vi "FT10_Semi-Auto Tester.vi"(7 "Read/ Write":T9, 8 "Error In":errorcluster, 10 "Semi-Auto Cluster in":T1 {"Power Level" format="%.1f"}, 11 "Path":path=path "FT10_rev2/Semi-Auto Commands.csv") -> (0 "Error Out":errorcluster, 2 "Semi-Auto Cluster out":T1 {"Power Level" format="%.1f"}, 3 "Semi-Auto 2-D Array out":T8)   [LabVIEW 2015]
doc: "READ = read CSV at specified path and pass commands out to be executed if user chooses.\n\nWRITE = write the cluster array to the specified CSV filepath. Then pass commands out to be executed if user chooses."
uses:
  LV2024/NI Online Practice/CLD Practice/cld_success_package/Preparation_Materials/CLD 6/CLD 6 CSV file enum.ctl
  Controls/Control_Semi-Auto 2-D Array.ctl
  Controls/Control_Semi-Auto Cluster Array.ctl
  Controls/Control_Semi-Auto Cluster.ctl
  Controls/Control_Semi-Auto Unitherm Load.ctl
  Controls/Control_Semi-Auto Port.ctl
  Controls/Control_Semi-Auto Mode.ctl
  Controls/Control_Semi-Auto Power Level.ctl
  Controls/Control_Semi-Auto Activation Duration.ctl
  Controls/Control_Semi-Auto 1-D Array.ctl
  <vilib>/Utility/file.llb/Read Delimited Spreadsheet (string).vi
  <vilib>/Utility/file.llb/Write Delimited Spreadsheet (string).vi
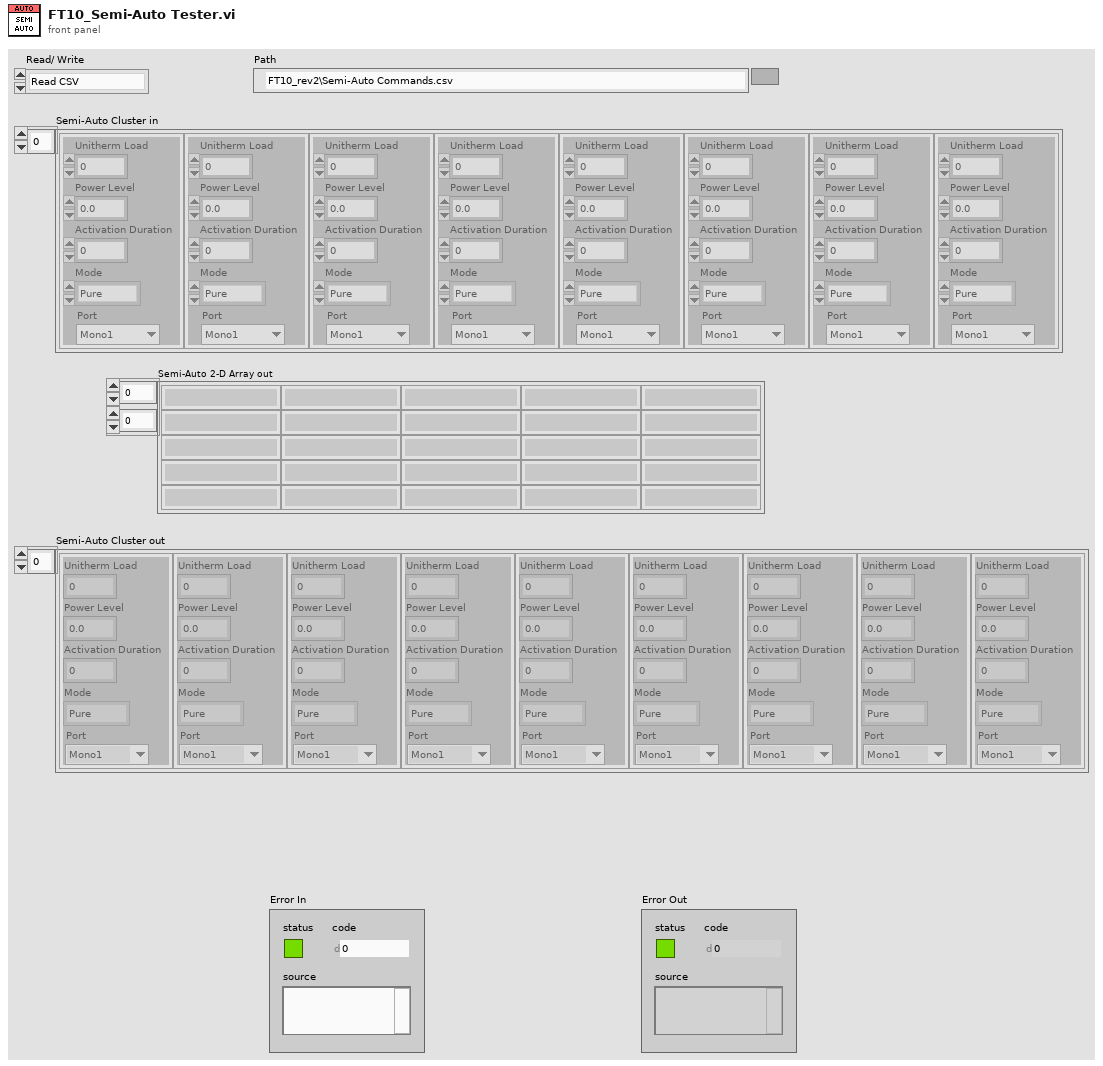
[diagram p1: front panel]
types:
  T1 = typedef "Control_Semi-Auto Cluster Array.ctl" = T2[]
  T2 = typedef "Control_Semi-Auto Cluster.ctl" = cluster{"Unitherm Load":T3, "Port":T4, "Mode":T5, "Power Level":T6, "Activation Duration":T7}
  T3 = typedef "Control_Semi-Auto Unitherm Load.ctl" = i32
  T4 = typedef "Control_Semi-Auto Port.ctl" = enum16{"Mono1", "Mono2", "Bipolar", "Ligasure", "Error"}
  T5 = typedef "Control_Semi-Auto Mode.ctl" = enum16{"Pure", "Blend", "Spray", "Fulgerate", "Standard", "Macro", "Precision", "Ligasure", "Error"}
  T6 = typedef "Control_Semi-Auto Power Level.ctl" = dbl
  T7 = typedef "Control_Semi-Auto Activation Duration.ctl" = i32
  T8 = typedef "Control_Semi-Auto 2-D Array.ctl" = string[][]
  T9 = typedef "CLD 6 CSV file enum.ctl" = enum16{"Read CSV", "Write CSV"}
  T10 = typedef "Control_Semi-Auto 1-D Array.ctl" = string[]
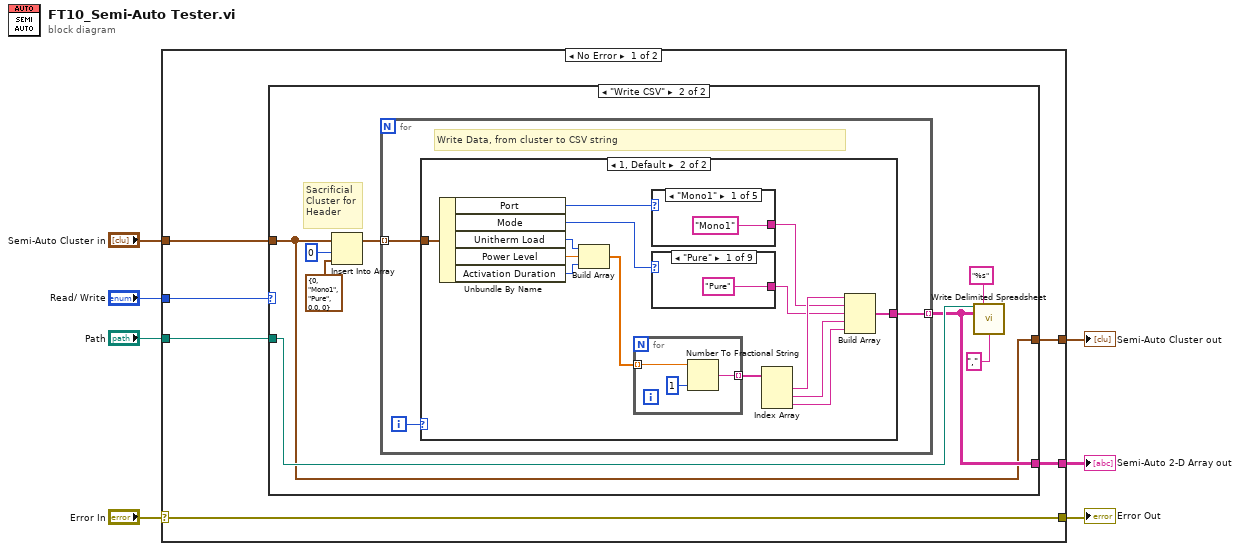
[diagram p0: block diagram]
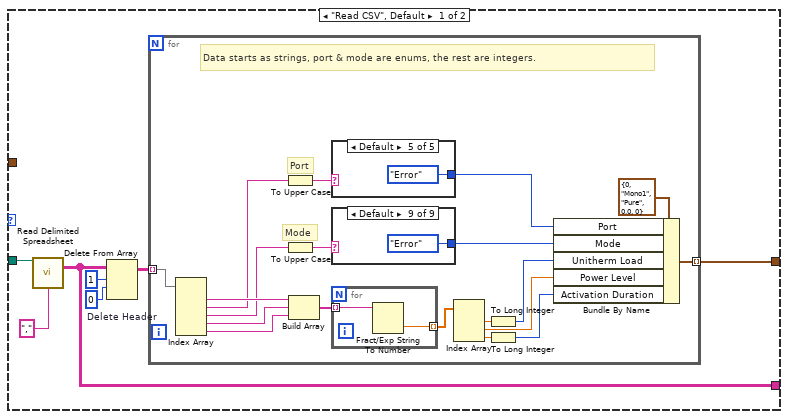
[diagram p2: hidden frame]
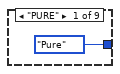
[diagram p3: hidden frame]
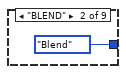
[diagram p4: hidden frame]
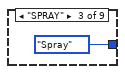
[diagram p5: hidden frame]
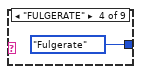
[diagram p6: hidden frame]
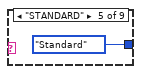
[diagram p7: hidden frame]
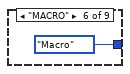
[diagram p8: hidden frame]
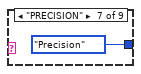
[diagram p9: hidden frame]
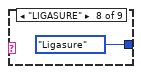
[diagram p10: hidden frame]
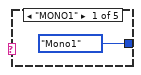
[diagram p11: hidden frame]
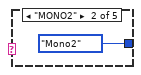
[diagram p12: hidden frame]
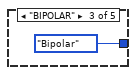
[diagram p13: hidden frame]
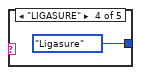
[diagram p14: hidden frame]
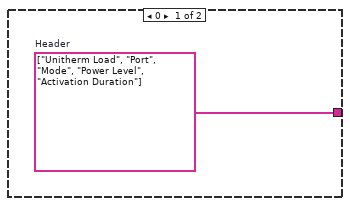
[diagram p15: hidden frame]
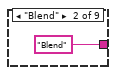
[diagram p16: hidden frame]
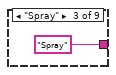
[diagram p17: hidden frame]
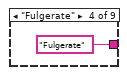
[diagram p18: hidden frame]
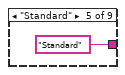
[diagram p19: hidden frame]
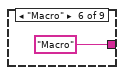
[diagram p20: hidden frame]
diagram:
  n1 = case shown="No Error" "Error In" {
    selector: "Error In" -> [w10 w101]
    tunnel: [w13 T1 []] -> w2
    tunnel: "Path" -> [w8 _]
    tunnel: "Read/ Write" -> [w12 _]
    tunnel: "Semi-Auto Cluster in" -> [w11 _]
    tunnel: [w10 w101] -> w4
    tunnel: [w9 string[][] [] ("all rows")] -> w3
    frame No Error {
      n2 = case shown="\"Write CSV\"" w12 {
        tunnel: w8 -> [w19 w62]
        tunnel: [w20 w59] -> w13
        tunnel: w11 -> [_ w59]
        tunnel: [w17 w60] -> w9
        frame "Read CSV", Default {
          n3 = call-poly <vilib>:"Read Delimited Spreadsheet.vi"("file path (dialog if empty)"=w19, "delimiter (\\t)"="," ("delimiter (\\t)")) -> ("all rows"=w17:string[][])  [unwired: 8 in, 5 out]
          n4 = Delete From Array "Delete Header"(array=w17, length=1, index (row)=0) -> (array with subset deleted=w16:string[][])  [unwired: 1 in, 1 out]
          n5 = for {
            tunnel: w16 -> [w39] mode=indexing
            tunnel: [w21] -> w20 mode=indexing
            # "Mode"
            # "Port"
            # "Data starts as strings, port & mode are enums, the rest are integers."
            n6 = Index Array "Index Array"(array=w39) -> (element #1=w38:string, element #2=w34:string, element #3=w33:string, element #4=w37:string, element #5=w36:string)  [unwired: 5 in]
            n7 = To Upper Case(1:w34) -> (0:w28:string)
            n8 = To Upper Case(1:w33) -> (0:w29:string)
            n9 = Build Array(w38, w37, w36) -> (w32:string[])
            n10 = case shown="Default" w28 {
              tunnel: [Control_Semi-Auto_Port."Mono1" ("Port") Control_Semi-Auto_Port."Mono2" ("Port") Control_Semi-Auto_Port."Bipolar" ("Port") Control_Semi-Auto_Port."Ligasure" ("Port") Control_Semi-Auto_Port."Error" ("Port")] -> w27
              frame "MONO1" {
              }
              frame "MONO2" {
              }
              frame "BIPOLAR" {
              }
              frame "LIGASURE" {
              }
              frame Default {
              }
            }
            n11 = case shown="Default" w29 {
              tunnel: [Control_Semi-Auto_Mode."Pure" ("Mode") Control_Semi-Auto_Mode."Blend" ("Mode") Control_Semi-Auto_Mode."Spray" ("Mode") Control_Semi-Auto_Mode."Fulgerate" ("Mode") Control_Semi-Auto_Mode."Standard" ("Mode") Control_Semi-Auto_Mode."Macro" ("Mode") Control_Semi-Auto_Mode."Precision" ("Mode") Control_Semi-Auto_Mode."Ligasure" ("Mode") Control_Semi-Auto_Mode."Error" ("Mode")] -> w26
              frame "PURE" {
              }
              frame "BLEND" {
              }
              frame "SPRAY" {
              }
              frame "FULGERATE" {
              }
              frame "STANDARD" {
              }
              frame "MACRO" {
              }
              frame "PRECISION" {
              }
              frame "LIGASURE" {
              }
              frame Default {
              }
            }
            n12 = for {
              tunnel: w32 -> [w55] mode=indexing
              tunnel: [w54] -> w31 mode=indexing
              n13 = Fract/Exp String To Number(string=w55) -> (number=w54:dbl)  [unwired: 3 in, 1 out]
            }
            n14 = Index Array "Index Array"(array=w31) -> (element #1=w24:dbl, element #2=w25:dbl, element #3=w30:dbl)  [unwired: 3 in]
            n15 = To Long Integer(number=w24) -> (32bit integer=w23:i32)
            n16 = To Long Integer(number=w30) -> (32bit integer=w22:i32)
            n17 = Bundle By Name(cluster=T2 {"Unitherm Load"=0, "Port"=enum."Mono1", "Mode"=enum."Pure", "Power Level"=0.0, "Activation Duration"=0}, "Port"=w27, "Mode"=w26, "Unitherm Load"=w23, "Power Level"=w25, "Activation Duration"=w22) -> (w21:T2)
          }
        }
        frame "Write CSV" {
          # "Sacrificial\nCluster for\nHeader"
          n18 = Insert Into Array(array=w59, index=0, new element=T2 {"Unitherm Load"=0, "Port"=enum."Mono1", "Mode"=enum."Pure", "Power Level"=0.0, "Activation Duration"=0}) -> (w56:T1)
          n19 = for {
            tunnel: w56 -> [w66] mode=indexing
            tunnel: [w65] -> w60 mode=indexing
            i -> [w64]
            # "Write Data, from cluster to CSV string"
            n20 = case shown="1, Default" w64 {
              tunnel: w66 -> [_ w81]
              tunnel: [w67 w72] -> w65
              frame 0 {
                w67 = T10 ["Unitherm Load", "Port", "Mode", "Power Level", "Activation Duration"]  # Header
              }
              frame 1, Default {
                n21 = Unbundle By Name(w81) -> ("Port"=w71:T4, "Mode"=w70:T5, "Unitherm Load"=w78:T3, "Power Level"=w79:T6, "Activation Duration"=w80:T7)
                n22 = Build Array(w78, w79, w80) -> (w77:T6[])
                n23 = for {
                  tunnel: w77 -> [w97] mode=indexing
                  tunnel: [w96] -> w76 mode=indexing
                  n24 = Number To Fractional String(number=w97, precision (6)=i16 1) -> (F-format string=w96:string)  [unwired: 2 in]
                }
                n25 = case shown="\"Mono1\"" w71 {
                  tunnel: ["Mono1" "Mono2" "Bipolar" "Ligasure" "Error"] -> w68
                  frame "Mono1" {
                  }
                  frame "Mono2" {
                  }
                  frame "Bipolar" {
                  }
                  frame "Ligasure" {
                  }
                  frame Default {
                  }
                }
                n26 = case shown="\"Pure\"" w70 {
                  tunnel: ["Pure" "Blend" "Spray" "Fulgerate" "Standard" "Macro" "Precision" "Ligasure" "Error"] -> w69
                  frame "Pure" {
                  }
                  frame "Blend" {
                  }
                  frame "Spray" {
                  }
                  frame "Fulgerate" {
                  }
                  frame "Standard" {
                  }
                  frame "Macro" {
                  }
                  frame "Precision" {
                  }
                  frame "Ligasure" {
                  }
                  frame Default {
                  }
                }
                n27 = Index Array(array=w76) -> (element #1=w75:string, element #2=w74:string, element #3=w73:string)  [unwired: 3 in]
                n28 = Build Array(w75, w68, w69, w74, w73) -> (w72:string[])
              }
            }
          }
          n29 = call-poly <vilib>:"Write Delimited Spreadsheet.vi"("file path (dialog if empty)"=w62, "format (%s)"="%s", "2D data"=w60, "delimiter (\\t)"="," ("delimiter (\\t)")) -> ()  [unwired: 10 in, 2 out]
        }
      }
    }
    frame Error {
    }
  }
  "Error Out" <- w4
  "Semi-Auto 2-D Array out" <- w3
  "Semi-Auto Cluster out" <- w2
